vi "Read Counter Control Register.vi"(8 "error in (no error)":errorcluster, 11 "DG Number":i32) -> (0 "error out":errorcluster, 3 "Count":u32)   [LabVIEW 2009, in "POLARIS BME DG.lvlib"]
doc: "unsigned long ReadCounterControlRegister(long DG_Number);"
uses:
  POLARIS BME DG.lvlib
  BME DLL/DelayGenerator.dll
panel:
  # "NOTICE -- YOU MUST LEAVE THIS NOTICE IN PLACE.  PER THE TERMS OF THE LICENSE BELOW, YOU MAY SUBLICENSE THIS SOFTWARE \nIN ANY WAY THAT DOES NOT CONFLICT WITH THIS LICENSE.\n\n### BSD License (http://www.opensource.org/licenses/bsd-license.php) Begin ###\n \nCopyright (c) 2011, Applied Energetics, http://www.appliedenergetics.com,\n                               Richard Schwerdtfeger, <rschwerdtfeger@appliedenergetics.com>\n\nAll rights reserved.\n\nRedistribution and use in source and binary forms, with or without modification, are permitted provided that the \nfollowing conditions are met:\n\n    * Redistributions of source code must retain the above copyright notice, this list of conditions and the following disclaimer.\n    * Redistributions in binary form must reproduce the above copyright notice, this list of conditions and the following disclaimer \n       in the documentation and/or other materials provided with the distribution.\n    * Neither the name of Richard Schwerdtfeger, Applied Energetics, Inc., nor the names of its contributors may be used to \n       endorse or promote products derived from this software without specific prior written permission.\n\nTHIS SOFTWARE IS PROVIDED BY THE COPYRIGHT HOLDERS AND CONTRIBUTORS \"AS IS\" AND ANY EXPRESS OR IMPLIED WARRANTIES, \nINCLUDING, BUT NOT LIMITED TO, THE IMPLIED WARRANTIES OF MERCHANTABILITY AND FITNESS FOR A PARTICULAR PURPOSE ARE \nDISCLAIMED. IN NO EVENT SHALL THE COPYRIGHT OWNER OR CONTRIBUTORS BE LIABLE FOR ANY DIRECT, INDIRECT, INCIDENTAL,\n SPECIAL, EXEMPLARY, OR CONSEQUENTIAL DAMAGES (INCLUDING, BUT NOT LIMITED TO, PROCUREMENT OF SUBSTITUTE GOODS OR \nSERVICES; LOSS OF USE, DATA, OR PROFITS; OR BUSINESS INTERRUPTION) HOWEVER CAUSED AND ON ANY THEORY OF LIABILITY, \nWHETHER IN CONTRACT, STRICT LIABILITY, OR TORT (INCLUDING NEGLIGENCE OR OTHERWISE) ARISING IN ANY WAY OUT OF THE USE \nOF THIS SOFTWARE, EVEN IF ADVISED OF THE POSSIBILITY OF SUCH DAMAGE.\n\n### BSD License End ###"
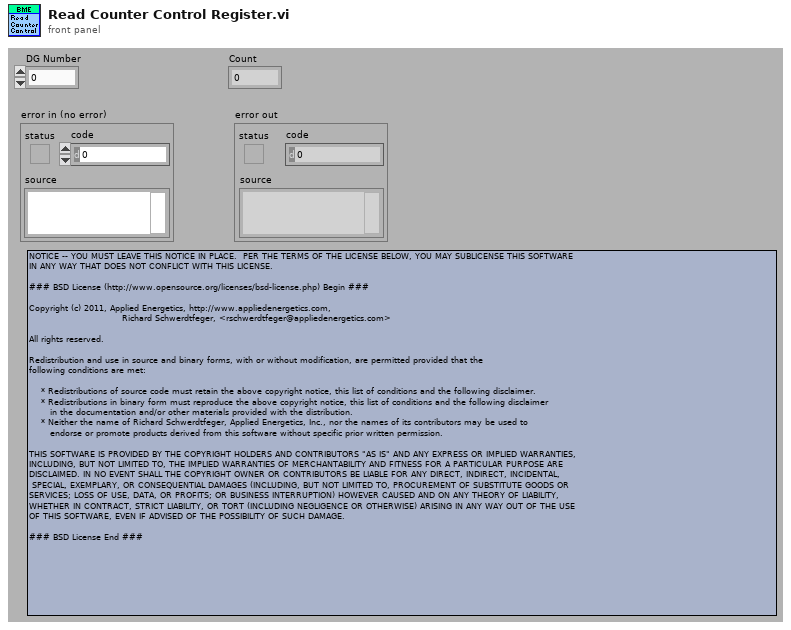
[diagram p1: front panel]
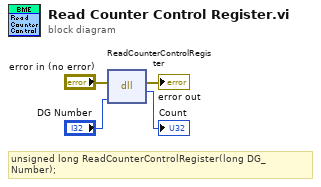
[diagram p0: block diagram]
diagram:
  # "unsigned long ReadCounterControlRegister(long DG_Number);"
  n1 = dll-call lib="C:/CS Framework/LVSCC/LV2009/GPL/Projects/cs-framework/CSClass/CSPOLARIS/POLARIS BME DG/BME DLL/DelayGenerator.*" fn="ReadCounterControlRegister"(error in="error in (no error)", "DG_Number"="DG Number") -> (error out=→"error out":errorcluster, →"Count":u32)  [unwired: 3 in, 1 out]
